vi "RM.addTreeEntries.vi"(8 "error in (no error)":errorcluster, 9 "Entries":T1(array[cluster]), 10 "Group Name":string="RIO Devices", 11 "TreeControl in":refnum<vi>) -> (0 "error out":errorcluster)   [LabVIEW 2016, in "FPGA Resource Manager.lvlib"]
uses:
  FPGA Resource Manager.lvlib
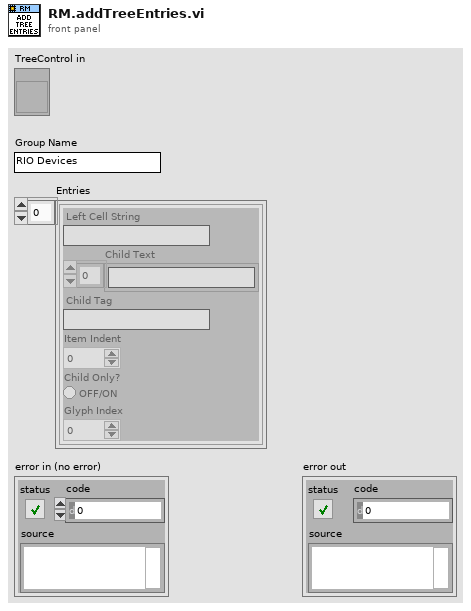
[diagram p1: front panel]
types:
  T1 = cluster{"Left Cell String":string, "Child Text":string[], "Child Tag":string, "Item Indent":i32, "Child Only?":bool, "Glyph Index":i32}[]
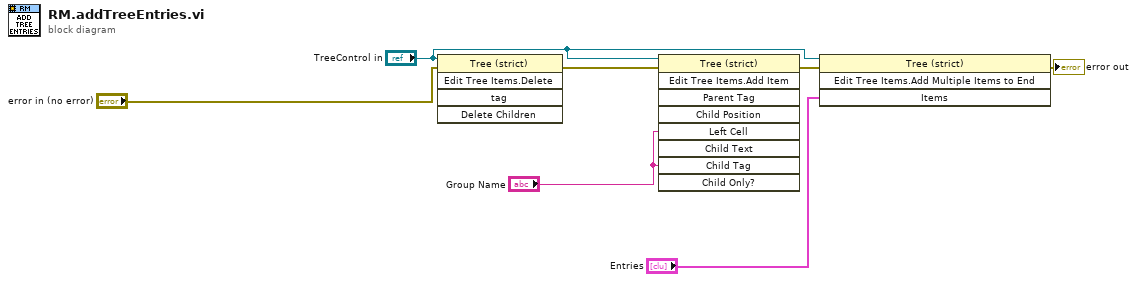
[diagram p0: block diagram]
diagram:
  n1 = invoke on="Invoke Node" class="Tree (strict)" method="Edit Tree Items.Delete"(reference="TreeControl in", error in="error in (no error)") -> (error out=w4:errorcluster)  [unwired: 3 in, 4 out]
  n2 = invoke on="Invoke Node" class="Tree (strict)" method="Edit Tree Items.Add Item"(reference="TreeControl in", error in=w4, "Left Cell"="Group Name", "Child Tag"="Group Name") -> (error out=w3:errorcluster)  [unwired: 5 in, 8 out]
  n3 = invoke on="Invoke Node" class="Tree (strict)" method="Edit Tree Items.Add Multiple Items to End"(reference="TreeControl in", error in=w3, "Items"="Entries") -> (error out=→"error out":errorcluster)  [unwired: 1 in, 3 out]
